vi "Write feedbackStatusInfo.vi"(8 "error in (no error)":errorcluster, 10 "feedbackStatusInfo":T1, 11 "RobotFeedback in":refnum<class "RobotFeedback.lvclass">) -> (0 "error out":errorcluster, 3 "RobotFeedback out":refnum<class "RobotFeedback.lvclass">)   [LabVIEW 2021, in "RobotFeedback.lvclass"]
uses:
  RobotFeedback.lvclass
  Game_class/feedbackStatusInfo.ctl
  RobotFeedback.lvclass/RobotFeedback.ctl
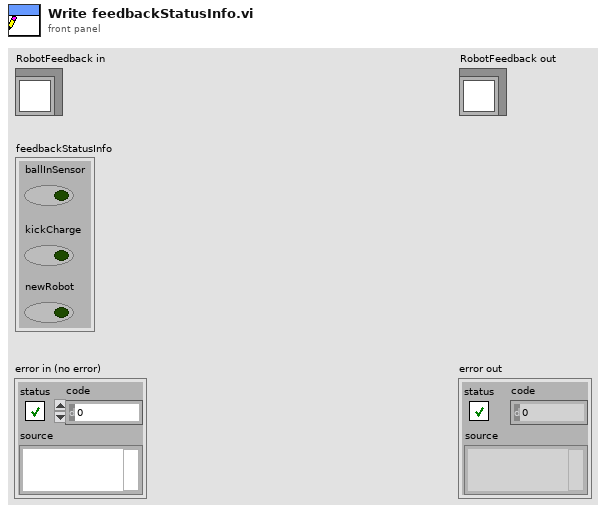
[diagram p1: front panel]
types:
  T1 = typedef "feedbackStatusInfo.ctl" = cluster{"ballInSensor":bool, "kickCharge":bool, "newRobot":bool}
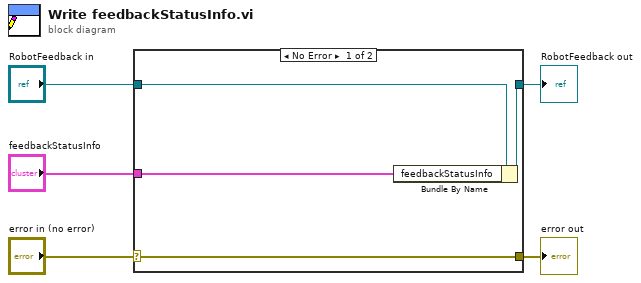
[diagram p0: block diagram]
diagram:
  n1 = case shown="No Error" "error in (no error)" {
    selector: "error in (no error)" -> [w9 w10]
    tunnel: [w9 w10] -> w4
    tunnel: [w7 w11] -> w2
    tunnel: "RobotFeedback in" -> [w8 w11]
    tunnel: "feedbackStatusInfo" -> [w6 _]
    frame No Error {
      n2 = Bundle By Name(cluster=w8, "feedbackStatusInfo"=w6) -> (w7:refnum<class "RobotFeedback.lvclass">)
    }
    frame Error {
    }
  }
  "error out" <- w4
  "RobotFeedback out" <- w2
